vi "Swap King in 1D Board.vi"(0 "1D Board":T1[](array[typedef]), 5 "King Index":i32, 7 "Cell Index":i32, 11 "error in (no error)":errorcluster) -> (4 "1D Board Out":T1[](array[typedef]), 15 "error out":errorcluster)   [LabVIEW 2014]
uses:
  Typedefs/Board Cell.ctl
  Typedefs/Cell Occupancy.ctl
  Dragon Tamers.lvlib
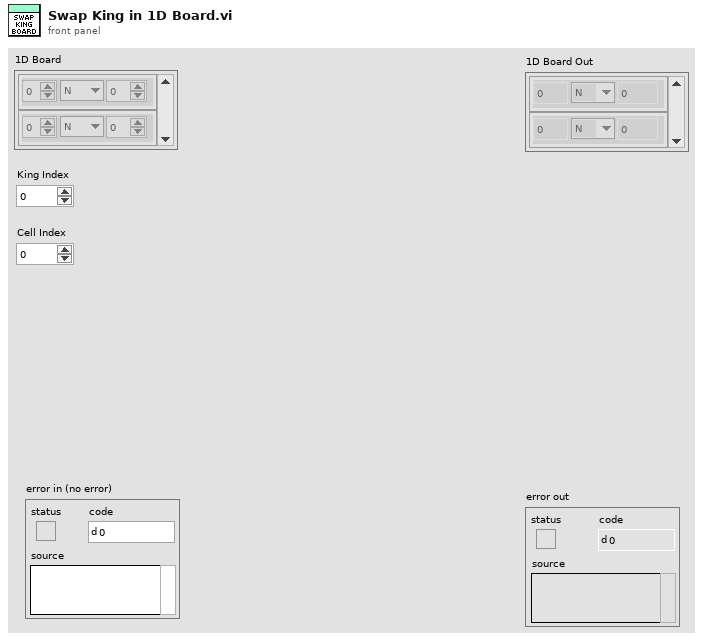
[diagram p1: front panel]
types:
  T1 = typedef "Dragon Tamers.lvlib/Board Cell.ctl" = cluster{"Team":i32, "Occu.":T2, "Count":i32}
  T2 = typedef "Dragon Tamers.lvlib/Cell Occupancy.ctl" = enum16{"N", "C", "K"}
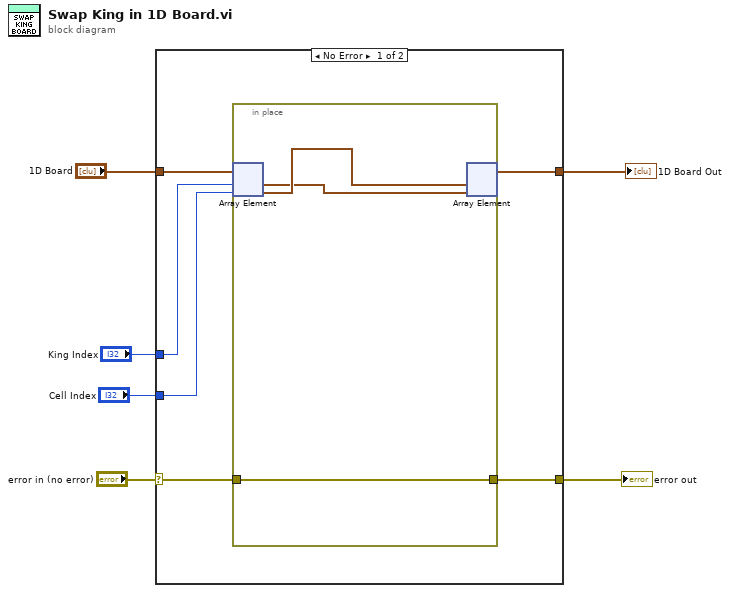
[diagram p0: block diagram]
diagram:
  n1 = case shown="No Error" "error in (no error)" {
    selector: "error in (no error)" -> [w7 w16]
    tunnel: [w8 w16] -> w5
    tunnel: "1D Board" -> [w12 _]
    tunnel: "King Index" -> [w11 _]
    tunnel: "Cell Index" -> [w10 _]
    tunnel: [w9 _] -> w1
    frame No Error {
      n2 = in-place {
        in-place-border: [w13] -> w8
        in-place-border: w7 -> [w13]
        n3 = in-place-array #1(w12, w11, w10) -> (w14:T1, w15:T1)
        n4 = in-place-array #1(w15, w14) -> (w9:T1[])  [unwired: 2 out]
      }
    }
    frame Error {
    }
  }
  "error out" <- w5
  "1D Board Out" <- w1
